vi "feeder_tester.vi"() -> ()   [LabVIEW 2012]
panel:
  out "Ready":bool
  in  "Shoot":bool
  out "CurrentAngle":dbl
  in  "Start Angle":dbl
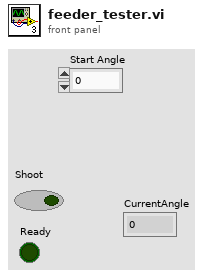
[diagram p1: front panel]
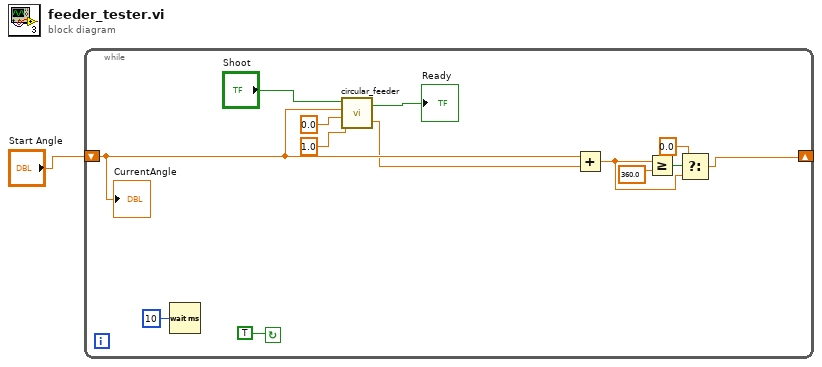
[diagram p0: block diagram]
diagram:
  n1 = while {
    shift-right: [w8] -> _
    shift-left: "Start Angle" -> [w5]
    stop <- TRUE continue-if-true
    n2 = Wait (ms)(milliseconds to wait=u32 10) -> ()  [unwired: 1 out]
    n3 = call "circular_feeder.vi"("Shoot"="Shoot", "Angle"=w5, "Stop Angle"=0.0, "Shooting Speed"=1.0) -> ("Ready"=→"Ready":bool, "Motor Voltage"=w4:dbl)  [unwired: 1 in]
    n4 = Add(x=w5, y=w4) -> (x+y=w11:dbl)
    n5 = Greater Or Equal?(x=w11, y=360.0) -> (x >= y?=w12:bool)
    n6 = Select(t=0.0, s=w12, f=w11) -> (s? t:f=w8:dbl)
    "CurrentAngle" <- w5
  }
